vi "Streamlines.vi"() -> ()   [LabVIEW 2011]
uses:
  <vilib>/Heliosphere Research LLC/Advanced Plotting Toolkit/Advanced Plotting Toolkit.lvlib
  <vilib>/Heliosphere Research LLC/Advanced Plotting Toolkit/typedefs/PlotColor.ctl
  <vilib>/Heliosphere Research LLC/Advanced Plotting Toolkit/api_core/NewPlotProperties.ctl
  <vilib>/Heliosphere Research LLC/Advanced Plotting Toolkit/properties/Line_Style.ctl
  <vilib>/Heliosphere Research LLC/Advanced Plotting Toolkit/properties/Line.ctl
  <vilib>/Heliosphere Research LLC/Advanced Plotting Toolkit/properties/Colormap_Map.ctl
  <vilib>/Heliosphere Research LLC/Advanced Plotting Toolkit/properties/Colormap_Scaling.ctl
  <vilib>/Heliosphere Research LLC/Advanced Plotting Toolkit/properties/Colormap.ctl
  <vilib>/Heliosphere Research LLC/Advanced Plotting Toolkit/api_plotting/StreamlineProperties.ctl
  <vilib>/Heliosphere Research LLC/Advanced Plotting Toolkit/properties/Display.ctl
  <vilib>/Heliosphere Research LLC/Advanced Plotting Toolkit/api_annotations/ShapeProperties.ctl
panel:
  in  "Colormap":T1=enum."White-Blue"
  in  "Arrow Size":dbl=1.0
  in  "Density":dbl=1.5
  out "Vector Plot":picture
  # "Streamlines"
  # "This VI demonstrates another way to visualize a vector field,\nusing streamlines.  Like VectorField.vi, provide a pair of 2D\narrays, giving the X and Y components of a vector field across\nthe plane.  Streamlines are automatically generated, depicting\nthe direction and density of the flow.\n\nThis example shows fluid flow past a cylinder.  Like\nVectorField.vi, the streamlines may be colormapped by\nproviding a 2D array of values.  In this case, we use the\nmagnitude of the vector field, which represents the flow\nspeed.\n\nThe number of streamlines may be increased via a density\nvalue. High values may result in reduced performance.\nEach streamline also has an arrow, whose size can be changed\nvia the property cluster."
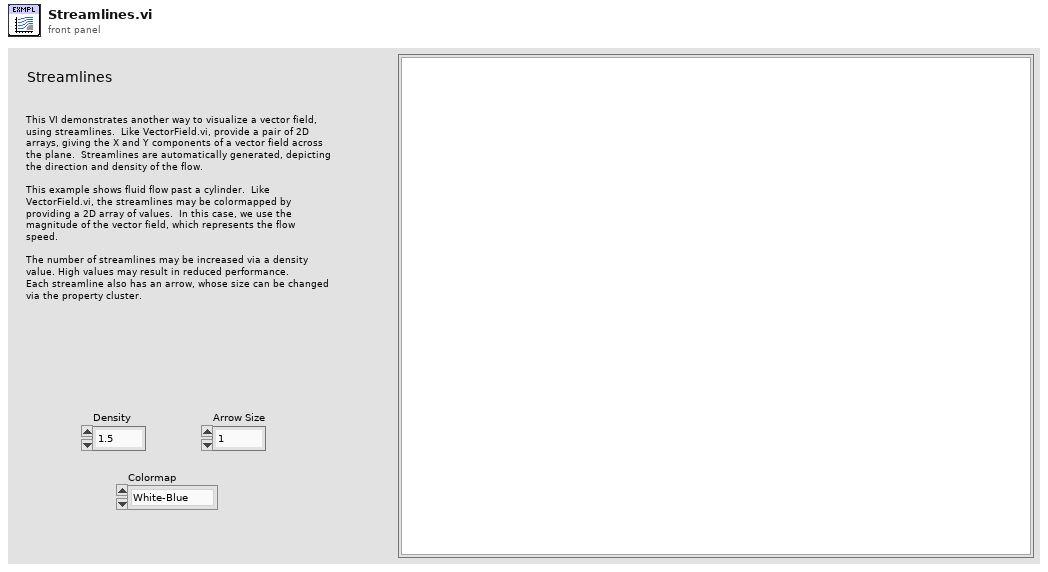
[diagram p1: front panel]
types:
  T1 = typedef "Advanced Plotting Toolkit.lvlib/Colormap_Map.ctl" = enum16{"Automatic", "Rainbow", "Hot and Cold", "White-Black", "White-Blue", "White-Green", "White-Red", "Fire", "Water", "Earth", "Air", "Pastel", "Banded", "Stepped"}
  T2 = typedef "Advanced Plotting Toolkit.lvlib/ShapeProperties.ctl" = cluster{"Color":T3, "Line":T4, "Display":T6}
  T3 = typedef "Advanced Plotting Toolkit.lvlib/PlotColor.ctl" = u32
  T4 = typedef "Advanced Plotting Toolkit.lvlib/Line.ctl" = cluster{"Style":T5, "Color":T3, "Width":sgl}
  T5 = typedef "Advanced Plotting Toolkit.lvlib/Line_Style.ctl" = enum16{"Automatic", "Solid", "Dashed", "Dotted", "Dash-dot", "Invisible"}
  T6 = typedef "Advanced Plotting Toolkit.lvlib/Display.ctl" = cluster{"Alpha":dbl, "Z Order":dbl}
  T7 = typedef "Advanced Plotting Toolkit.lvlib/StreamlineProperties.ctl" = cluster{"Density":dbl, "Arrow Size":dbl, "Line":T4, "Colormap":T8}
  T8 = typedef "Advanced Plotting Toolkit.lvlib/Colormap.ctl" = cluster{"Map":T1, "Value Min":dbl, "Value Max":dbl, "Scaling":T9, "Reverse":bool}
  T9 = typedef "Advanced Plotting Toolkit.lvlib/Colormap_Scaling.ctl" = enum16{"Default"}
  T10 = typedef "Advanced Plotting Toolkit.lvlib/NewPlotProperties.ctl" = cluster{"Background Color":T3, "Axis Background":T3, "Left Margin":dbl, "Right Margin":dbl, "Bottom Margin":dbl, "Top Margin":dbl, "Aspect Ratio":dbl}
  T11 = typedef "Advanced Plotting Toolkit.lvlib/PlotID.ctl" = i32
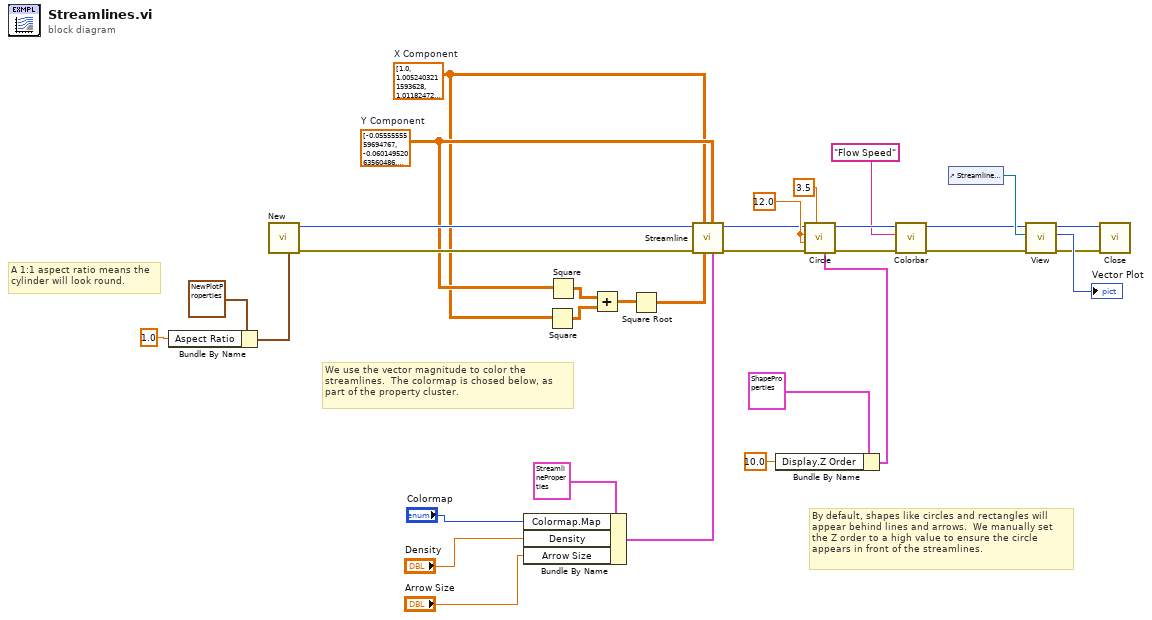
[diagram p0: block diagram]
diagram:
  w13 = 12.0 ("X Position")
  w21 = sgl[][] [[1.0, 1.0052403, 1.0118247, 1.0199112, 1.0295858, 1.0408064, 1.0533333, 1.0666643, 1.08, 1.0922722, 1.1022644, 1.1088228, 1.1111112, 1.1088228, 1.1022644, 1.0922722, 1.08, 1.0666643, 1.0533333, 1.0408064, 1.0295858, 1.0199112, 1.0118247, 1.0052403, 1.0], [0.9947597, 1.0, 1.0068794, 1.0156847, 1.0266472, 1.0398616, 1.0551747, 1.0720586, 1.0895092, 1.1060355, 1.119808, 1.1289976, 1.1322314, 1.1289976, 1.119808, 1.1060355, 1.0895092, 1.0720586, 1.0551747, 1.0398616, 1.0266472, 1.0156847, 1.0068794, 1.0, 0.9947597], [0.9881752, 0.99312055, 1.0, 1.0092794, 1.0214158, 1.0367551, 1.0553633, 1.0768, 1.099881, 1.1225486, 1.1420119, 1.1552789, 1.16, 1.1552789, 1.1420119, 1.1225486, 1.099881, 1.0768, 1.0553633, 1.0367551, 1.0214158, 1.0092794, 1.0, 0.99312055, 0.9881752], [0.9800889, 0.9843153, 0.9907207, 1.0, 1.012937, 1.0302958, 1.0525969, 1.0797436, 1.1105325, 1.1422222, 1.170519, 1.1903629, 1.1975309, 1.1903629, 1.170519, 1.1422222, 1.1105325, 1.0797436, 1.0525969, 1.0302958, 1.012937, 1.0, 0.9907207, 0.9843153, 0.9800889], [0.9704142, 0.9733528, 0.9785842, 0.987063, 1.0, 1.0187955, 1.0448, 1.0787779, 1.12, 1.1651342, 1.2076125, 1.2385799, 1.25, 1.2385799, 1.2076125, 1.1651342, 1.12, 1.0787779, 1.0448, 1.0187955, 1.0, 0.987063, 0.9785842, 0.9733528, 0.9704142], [0.9591935, 0.9601384, 0.9632449, 0.96970415, 0.98120445, 1.0, 1.0287889, 1.0701241, 1.1249704, 1.1902497, 1.2563189, 1.3072, 1.3265306, 1.3072, 1.2563189, 1.1902497, 1.1249704, 1.0701241, 1.0287889, 1.0, 0.98120445, 0.96970415, 0.9632449, 0.9601384, 0.9591935], [0.94666666, 0.94482535, 0.9446367, 0.947403, 0.9552, 0.9712111, 1.0, 1.0472991, 1.1183432, 1.2133334, 1.32, 1.4090577, 1.4444444, 1.4090577, 1.32, 1.2133334, 1.1183432, 1.0472991, 1.0, 0.9712111, 0.9552, 0.947403, 0.9446367, 0.94482535, 0.94666666], [0.93333566, 0.92794144, 0.9232, 0.9202563, 0.9212221, 0.92987585, 0.9527009, 1.0, 1.0856633, 1.2214533, 1.3995243, 1.5680473, 1.64, 1.5680473, 1.3995243, 1.2214533, 1.0856633, 1.0, 0.9527009, 0.92987585, 0.9212221, 0.9202563, 0.9232, 0.92794144, 0.93333566], [0.92, 0.9104907, 0.9001189, 0.88946754, 0.88, 0.87502956, 0.8816568, 0.9143367, 1.0, 1.1792, 1.48, 1.8304498, 0.0, 1.8304498, 1.48, 1.1792, 1.0, 0.9143367, 0.8816568, 0.87502956, 0.88, 0.88946754, 0.9001189, 0.9104907, 0.92], [0.9077278, 0.89396447, 0.8774514, 0.8577778, 0.8348658, 0.8097503, 0.7866667, 0.7785467, 0.8208, 1.0, 0.0, 0.0, 0.0, 0.0, 0.0, 1.0, 0.8208, 0.7785467, 0.7866667, 0.8097503, 0.8348658, 0.8577778, 0.8774514, 0.89396447, 0.9077278], [0.8977356, 0.880192, 0.8579882, 0.82948095, 0.79238755, 0.743681, 0.68, 0.6004756, 0.52, 0.0, 0.0, 0.0, 0.0, 0.0, 0.0, 0.0, 0.52, 0.6004756, 0.68, 0.743681, 0.79238755, 0.82948095, 0.8579882, 0.880192, 0.8977356], [0.8911772, 0.87100244, 0.8447211, 0.8096371, 0.76142013, 0.6928, 0.5909423, 0.43195266, 0.16955018, 0.0, 0.0, 0.0, 0.0, 0.0, 0.0, 0.0, 0.16955018, 0.43195266, 0.5909423, 0.6928, 0.76142013, 0.8096371, 0.8447211, 0.87100244, 0.8911772], [0.8888889, 0.8677686, 0.84, 0.80246913, 0.75, 0.67346936, 0.5555556, 0.36, 0.0, 0.0, 0.0, 0.0, 0.0, 0.0, 0.0, 0.0, 0.0, 0.36, 0.5555556, 0.67346936, 0.75, 0.80246913, 0.84, 0.8677686, 0.8888889], [0.8911772, 0.87100244, 0.8447211, 0.8096371, 0.76142013, 0.6928, 0.5909423, 0.43195266, 0.16955018, 0.0, 0.0, 0.0, 0.0, 0.0, 0.0, 0.0, 0.16955018, 0.43195266, 0.5909423, 0.6928, 0.76142013, 0.8096371, 0.8447211, 0.87100244, 0.8911772], [0.8977356, 0.880192, 0.8579882, 0.82948095, 0.79238755, 0.743681, 0.68, 0.6004756, 0.52, 0.0, 0.0, 0.0, 0.0, 0.0, 0.0, 0.0, 0.52, 0.6004756, 0.68, 0.743681, 0.79238755, 0.82948095, 0.8579882, 0.880192, 0.8977356], [0.9077278, 0.89396447, 0.8774514, 0.8577778, 0.8348658, 0.8097503, 0.7866667, 0.7785467, 0.8208, 1.0, 0.0, 0.0, 0.0, 0.0, 0.0, 1.0, 0.8208, 0.7785467, 0.7866667, 0.8097503, 0.8348658, 0.8577778, 0.8774514, 0.89396447, 0.9077278], [0.92, 0.9104907, 0.9001189, 0.88946754, 0.88, 0.87502956, 0.8816568, 0.9143367, 1.0, 1.1792, 1.48, 1.8304498, 0.0, 1.8304498, 1.48, 1.1792, 1.0, 0.9143367, 0.8816568, 0.87502956, 0.88, 0.88946754, 0.9001189, 0.9104907, 0.92], [0.93333566, 0.92794144, 0.9232, 0.9202563, 0.9212221, 0.92987585, 0.9527009, 1.0, 1.0856633, 1.2214533, 1.3995243, 1.5680473, 1.64, 1.5680473, 1.3995243, 1.2214533, 1.0856633, 1.0, 0.9527009, 0.92987585, 0.9212221, 0.9202563, 0.9232, 0.92794144, 0.93333566], [0.94666666, 0.94482535, 0.9446367, 0.947403, 0.9552, 0.9712111, 1.0, 1.0472991, 1.1183432, 1.2133334, 1.32, 1.4090577, 1.4444444, 1.4090577, 1.32, 1.2133334, 1.1183432, 1.0472991, 1.0, 0.9712111, 0.9552, 0.947403, 0.9446367, 0.94482535, 0.94666666], [0.9591935, 0.9601384, 0.9632449, 0.96970415, 0.98120445, 1.0, 1.0287889, 1.0701241, 1.1249704, 1.1902497, 1.2563189, 1.3072, 1.3265306, 1.3072, 1.2563189, 1.1902497, 1.1249704, 1.0701241, 1.0287889, 1.0, 0.98120445, 0.96970415, 0.9632449, 0.9601384, 0.9591935], [0.9704142, 0.9733528, 0.9785842, 0.987063, 1.0, 1.0187955, 1.0448, 1.0787779, 1.12, 1.1651342, 1.2076125, 1.2385799, 1.25, 1.2385799, 1.2076125, 1.1651342, 1.12, 1.0787779, 1.0448, 1.0187955, 1.0, 0.987063, 0.9785842, 0.9733528, 0.9704142], [0.9800889, 0.9843153, 0.9907207, 1.0, 1.012937, 1.0302958, 1.0525969, 1.0797436, 1.1105325, 1.1422222, 1.170519, 1.1903629, 1.1975309, 1.1903629, 1.170519, 1.1422222, 1.1105325, 1.0797436, 1.0525969, 1.0302958, 1.012937, 1.0, 0.9907207, 0.9843153, 0.9800889], [0.9881752, 0.99312055, 1.0, 1.0092794, 1.0214158, 1.0367551, 1.0553633, 1.0768, 1.099881, 1.1225486, 1.1420119, 1.1552789, 1.16, 1.1552789, 1.1420119, 1.1225486, 1.099881, 1.0768, 1.0553633, 1.0367551, 1.0214158, 1.0092794, 1.0, 0.99312055, 0.9881752], [0.9947597, 1.0, 1.0068794, 1.0156847, 1.0266472, 1.0398616, 1.0551747, 1.0720586, 1.0895092, 1.1060355, 1.119808, 1.1289976, 1.1322314, 1.1289976, 1.119808, 1.1060355, 1.0895092, 1.0720586, 1.0551747, 1.0398616, 1.0266472, 1.0156847, 1.0068794, 1.0, 0.9947597], [1.0, 1.0052403, 1.0118247, 1.0199112, 1.0295858, 1.0408064, 1.0533333, 1.0666643, 1.08, 1.0922722, 1.1022644, 1.1088228, 1.1111112, 1.1088228, 1.1022644, 1.0922722, 1.08, 1.0666643, 1.0533333, 1.0408064, 1.0295858, 1.0199112, 1.0118247, 1.0052403, 1.0]]  # X Component
  w22 = sgl[][] [[-0.055555556, -0.06014952, -0.06449879, -0.06826667, -0.07100592, -0.07216301, -0.07111111, -0.06722454, -0.06, -0.04921184, -0.03506209, -0.018263971, 0.0, 0.018263971, 0.03506209, 0.04921184, 0.06, 0.06722454, 0.07111111, 0.07216301, 0.07100592, 0.06826667, 0.06449879, 0.06014952, 0.055555556], [-0.06014952, -0.0661157, -0.0720706, -0.077639446, -0.082279034, -0.08525951, -0.08568299, -0.08256709, -0.07501732, -0.062485207, -0.045056, -0.023649557, 0.0, 0.023649557, 0.045056, 0.062485207, 0.07501732, 0.08256709, 0.08568299, 0.08525951, 0.082279034, 0.077639446, 0.0720706, 0.0661157, 0.06014952], [-0.06449879, -0.0720706, -0.08, -0.08790941, -0.09518144, -0.10089636, -0.10380623, -0.1024, -0.09512485, -0.08080128, -0.0591716, -0.031369474, 0.0, 0.031369474, 0.0591716, 0.08080128, 0.09512485, 0.1024, 0.10380623, 0.10089636, 0.09518144, 0.08790941, 0.08, 0.0720706, 0.06449879], [-0.06826667, -0.077639446, -0.08790941, -0.09876543, -0.10958383, -0.11928994, -0.12623274, -0.1281595, -0.122435965, -0.10666667, -0.07972319, -0.04283165, 0.0, 0.04283165, 0.07972319, 0.10666667, 0.122435965, 0.1281595, 0.12623274, 0.11928994, 0.10958383, 0.09876543, 0.08790941, 0.077639446, 0.06826667], [-0.07100592, -0.082279034, -0.09518144, -0.10958383, -0.125, -0.14033988, -0.1536, -0.16159576, -0.16, -0.1441171, -0.11072665, -0.060591716, 0.0, 0.060591716, 0.11072665, 0.1441171, 0.16, 0.16159576, 0.1536, 0.14033988, 0.125, 0.10958383, 0.09518144, 0.082279034, 0.07100592], [-0.07216301, -0.08525951, -0.10089636, -0.11928994, -0.14033988, -0.1632653, -0.18602076, -0.20452885, -0.212071, -0.19976218, -0.15948737, -0.0896, 0.0, 0.0896, 0.15948737, 0.19976218, 0.212071, 0.20452885, 0.18602076, 0.1632653, 0.14033988, 0.11928994, 0.10089636, 0.08525951, 0.07216301], [-0.07111111, -0.08568299, -0.10380623, -0.12623274, -0.1536, -0.18602076, -0.22222222, -0.25799516, -0.28402367, -0.28444445, -0.24, -0.14024836, 0.0, 0.14024836, 0.24, 0.28444445, 0.28402367, 0.25799516, 0.22222222, 0.18602076, 0.1536, 0.12623274, 0.10380623, 0.08568299, 0.07111111], [-0.06722454, -0.08256709, -0.1024, -0.1281595, -0.16159576, -0.20452885, -0.25799516, -0.32, -0.38072577, -0.4152249, -0.3804994, -0.2366864, 0.0, 0.2366864, 0.3804994, 0.4152249, 0.38072577, 0.32, 0.25799516, 0.20452885, 0.16159576, 0.1281595, 0.1024, 0.08256709, 0.06722454], [-0.06, -0.07501732, -0.09512485, -0.122435965, -0.16, -0.212071, -0.28402367, -0.38072577, -0.5, -0.6144, -0.64, -0.4429066, 0.0, 0.4429066, 0.64, 0.6144, 0.5, 0.38072577, 0.28402367, 0.212071, 0.16, 0.122435965, 0.09512485, 0.07501732, 0.06], [-0.04921184, -0.062485207, -0.08080128, -0.10666667, -0.1441171, -0.19976218, -0.28444445, -0.4152249, -0.6144, -0.8888889, 0.0, 0.0, 0.0, 0.0, 0.0, 0.8888889, 0.6144, 0.4152249, 0.28444445, 0.19976218, 0.1441171, 0.10666667, 0.08080128, 0.062485207, 0.04921184], [-0.03506209, -0.045056, -0.0591716, -0.07972319, -0.11072665, -0.15948737, -0.24, -0.3804994, -0.64, 0.0, 0.0, 0.0, 0.0, 0.0, 0.0, 0.0, 0.64, 0.3804994, 0.24, 0.15948737, 0.11072665, 0.07972319, 0.0591716, 0.045056, 0.03506209], [-0.018263971, -0.023649557, -0.031369474, -0.04283165, -0.060591716, -0.0896, -0.14024836, -0.2366864, -0.4429066, 0.0, 0.0, 0.0, 0.0, 0.0, 0.0, 0.0, 0.4429066, 0.2366864, 0.14024836, 0.0896, 0.060591716, 0.04283165, 0.031369474, 0.023649557, 0.018263971], [0.0, 0.0, 0.0, 0.0, 0.0, 0.0, 0.0, 0.0, 0.0, 0.0, 0.0, 0.0, 0.0, 0.0, 0.0, 0.0, 0.0, 0.0, 0.0, 0.0, 0.0, 0.0, 0.0, 0.0, 0.0], [0.018263971, 0.023649557, 0.031369474, 0.04283165, 0.060591716, 0.0896, 0.14024836, 0.2366864, 0.4429066, 0.0, 0.0, 0.0, 0.0, 0.0, 0.0, 0.0, -0.4429066, -0.2366864, -0.14024836, -0.0896, -0.060591716, -0.04283165, -0.031369474, -0.023649557, -0.018263971], [0.03506209, 0.045056, 0.0591716, 0.07972319, 0.11072665, 0.15948737, 0.24, 0.3804994, 0.64, 0.0, 0.0, 0.0, 0.0, 0.0, 0.0, 0.0, -0.64, -0.3804994, -0.24, -0.15948737, -0.11072665, -0.07972319, -0.0591716, -0.045056, -0.03506209], [0.04921184, 0.062485207, 0.08080128, 0.10666667, 0.1441171, 0.19976218, 0.28444445, 0.4152249, 0.6144, 0.8888889, 0.0, 0.0, 0.0, 0.0, 0.0, -0.8888889, -0.6144, -0.4152249, -0.28444445, -0.19976218, -0.1441171, -0.10666667, -0.08080128, -0.062485207, -0.04921184], [0.06, 0.07501732, 0.09512485, 0.122435965, 0.16, 0.212071, 0.28402367, 0.38072577, 0.5, 0.6144, 0.64, 0.4429066, 0.0, -0.4429066, -0.64, -0.6144, -0.5, -0.38072577, -0.28402367, -0.212071, -0.16, -0.122435965, -0.09512485, -0.07501732, -0.06], [0.06722454, 0.08256709, 0.1024, 0.1281595, 0.16159576, 0.20452885, 0.25799516, 0.32, 0.38072577, 0.4152249, 0.3804994, 0.2366864, 0.0, -0.2366864, -0.3804994, -0.4152249, -0.38072577, -0.32, -0.25799516, -0.20452885, -0.16159576, -0.1281595, -0.1024, -0.08256709, -0.06722454], [0.07111111, 0.08568299, 0.10380623, 0.12623274, 0.1536, 0.18602076, 0.22222222, 0.25799516, 0.28402367, 0.28444445, 0.24, 0.14024836, 0.0, -0.14024836, -0.24, -0.28444445, -0.28402367, -0.25799516, -0.22222222, -0.18602076, -0.1536, -0.12623274, -0.10380623, -0.08568299, -0.07111111], [0.07216301, 0.08525951, 0.10089636, 0.11928994, 0.14033988, 0.1632653, 0.18602076, 0.20452885, 0.212071, 0.19976218, 0.15948737, 0.0896, 0.0, -0.0896, -0.15948737, -0.19976218, -0.212071, -0.20452885, -0.18602076, -0.1632653, -0.14033988, -0.11928994, -0.10089636, -0.08525951, -0.07216301], [0.07100592, 0.082279034, 0.09518144, 0.10958383, 0.125, 0.14033988, 0.1536, 0.16159576, 0.16, 0.1441171, 0.11072665, 0.060591716, 0.0, -0.060591716, -0.11072665, -0.1441171, -0.16, -0.16159576, -0.1536, -0.14033988, -0.125, -0.10958383, -0.09518144, -0.082279034, -0.07100592], [0.06826667, 0.077639446, 0.08790941, 0.09876543, 0.10958383, 0.11928994, 0.12623274, 0.1281595, 0.122435965, 0.10666667, 0.07972319, 0.04283165, 0.0, -0.04283165, -0.07972319, -0.10666667, -0.122435965, -0.1281595, -0.12623274, -0.11928994, -0.10958383, -0.09876543, -0.08790941, -0.077639446, -0.06826667], [0.06449879, 0.0720706, 0.08, 0.08790941, 0.09518144, 0.10089636, 0.10380623, 0.1024, 0.09512485, 0.08080128, 0.0591716, 0.031369474, 0.0, -0.031369474, -0.0591716, -0.08080128, -0.09512485, -0.1024, -0.10380623, -0.10089636, -0.09518144, -0.08790941, -0.08, -0.0720706, -0.06449879], [0.06014952, 0.0661157, 0.0720706, 0.077639446, 0.082279034, 0.08525951, 0.08568299, 0.08256709, 0.07501732, 0.062485207, 0.045056, 0.023649557, 0.0, -0.023649557, -0.045056, -0.062485207, -0.07501732, -0.08256709, -0.08568299, -0.08525951, -0.082279034, -0.077639446, -0.0720706, -0.0661157, -0.06014952], [0.055555556, 0.06014952, 0.06449879, 0.06826667, 0.07100592, 0.07216301, 0.07111111, 0.06722454, 0.06, 0.04921184, 0.03506209, 0.018263971, 0.0, -0.018263971, -0.03506209, -0.04921184, -0.06, -0.06722454, -0.07111111, -0.07216301, -0.07100592, -0.06826667, -0.06449879, -0.06014952, -0.055555556]]  # Y Component
  # "By default, shapes like circles and rectangles will\nappear behind lines and arrows.  We manually set\nthe Z order to a high value to ensure the circle\nappears in front of the streamlines."
  # "We use the vector magnitude to color the\nstreamlines.  The colormap is chosed below, as\npart of the property cluster."
  # "A 1:1 aspect ratio means the\ncylinder will look round."
  n1 = Bundle By Name(cluster=T10 {"Background Color"=2147483647, "Axis Background"=2147483647, "Left Margin"=nan, "Right Margin"=nan, "Bottom Margin"=nan, "Top Margin"=nan, "Aspect Ratio"=nan} ("New Plot Properties"), "Aspect Ratio"=1.0) -> (w26:T10)
  n2 = call <vilib>:"New.vi"("Properties"=w26) -> ("error out"=w25:errorcluster, "Plot ID"=w29:T11)  [unwired: 9 in]
  n3 = Bundle By Name(cluster=T7 {"Density"=nan, "Arrow Size"=nan, "Line"={"Style"=enum."Automatic", "Color"=2147483647, "Width"=nan}, "Colormap"={"Map"=enum."Automatic", "Value Min"=nan, "Value Max"=nan, "Scaling"=enum."Default", "Reverse"=FALSE}} ("Streamline Properties"), "Colormap.Map"="Colormap", "Density"="Density", "Arrow Size"="Arrow Size") -> (w15:T7)
  n4 = Square(x=w21) -> (x^2=w18:sgl[][])
  n5 = Square(x=w22) -> (x^2=w19:sgl[][])
  n6 = Add(x=w19, y=w18) -> (x+y=w20:sgl[][])
  n7 = Square Root(x=w20) -> (sqrt(x)=w17:sgl[][])
  n8 = call <vilib>:"Streamline.vi"("Properties"=w15, "Y Vector Component"=w22, "Colormap Value"=w17, "X Vector Component"=w21, "error in (no error)"=w25, "Plot ID"=w29) -> ("error out"=w10:errorcluster, "Plot ID Out"=w11:T11)  [unwired: 4 in]
  n9 = Bundle By Name(cluster=T2 {"Color"=2147483647, "Line"={"Style"=enum."Automatic", "Color"=2147483647, "Width"=nan}, "Display"={"Alpha"=nan, "Z Order"=nan}} ("Shape Properties"), "Display.Z Order"=10.0) -> (w5:T2)
  n10 = call <vilib>:"Circle.vi"("Properties"=w5, "Radius"=3.5, "error in (no error)"=w10, "Y Position"=w13, "X Position"=w13, "Plot ID"=w11) -> ("error out"=w8:errorcluster, "Plot ID Out"=w9:T11)  [unwired: 4 in]
  n11 = call <vilib>:"Colorbar.vi"("error in (no error)"=w8, "Label"="Flow Speed", "Plot ID"=w9) -> ("error out"=w23:errorcluster, "Plot ID Out"=w24:T11)  [unwired: 7 in]
  n12 = control-ref of="Streamline Plot"() -> (w31:refnum<vi>)
  n13 = call <vilib>:"View.vi"("error in (no error)"=w23, "Ref for Sizing"=w31, "Plot ID"=w24) -> ("error out"=w1:errorcluster, "Picture"=→"Vector Plot":picture, "Plot ID Out"=w30:T11)  [unwired: 6 in]
  n14 = call <vilib>:"Close.vi"("error in (no error)"=w1, "Plot ID"=w30) -> ()  [unwired: 9 in, 1 out]
